vi "Inspect Tell.vi"(8 "Error in":errorcluster, 9 "Msg Attributes":refnum<data-value>, 10 "Alias":string, 11 "TEMPLATE Actor in":refnum<class "TEMPLATE Actor.lvclass">) -> (0 "Error out":errorcluster, 2 "Proceed To Tell":bool=TRUE, 3 "TEMPLATE Actor out":refnum<class "TEMPLATE Actor.lvclass">)   [LabVIEW 2020, in "_Template.lvlib" / "Templates.lvlib" / "TEMPLATE jettl Actor.lvlib" / "TEMPLATE Actor.lvlib" / "TEMPLATE Actor.lvclass"]
uses:
  TEMPLATE Actor.lvclass
  TEMPLATE Actor.lvclass/TEMPLATE Actor.ctl
  jettl/jettl/Actor/Actor.lvclass
  jettl/jettl/Msg/Msg.lvclass
  jettl/jettl/Refs/Refs.lvclass
  jettl/jettl/Relation.ctl
  jettl/jettl/jettl.lvlib
  jettl/jettl/Teller.ctl
  jettl/jettl/Msg Input/Msg Input.lvclass
  jettl/jettl/Msg Output/Msg Output.lvclass
  jettl/jettl/Msg Attributes.ctl
panel:
  # "This front panel should not be manipulated."
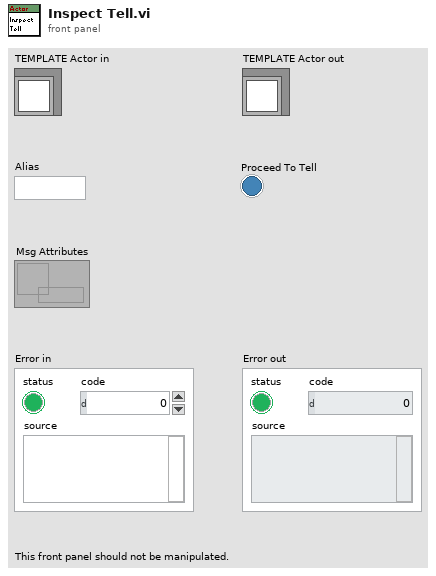
[diagram p1: front panel]
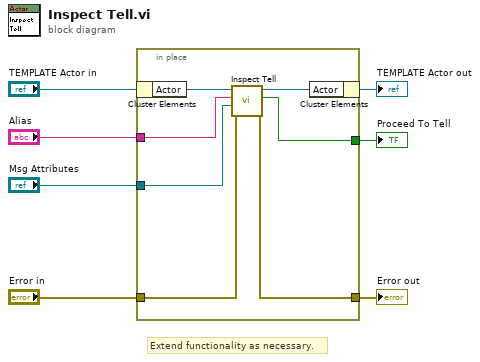
[diagram p0: block diagram]
diagram:
  # "Extend functionality as necessary."
  n1 = in-place {
    in-place-border: "Error in" -> [w11]
    in-place-border: "Msg Attributes" -> [w12]
    in-place-border: [w10] -> w3
    in-place-border: [w9] -> w2
    in-place-border: "Alias" -> [w8]
    n2 = in-place-cluster #1("TEMPLATE Actor in") -> ("Actor"=w14:refnum<data-value>)
    n3 = call-dynamic "Inspect Tell.vi"("Error in"=w11, "Msg Attributes"=w12, "Alias"=w8, "Actor in"=w14) -> ("Error out"=w10:errorcluster, "Proceed To Tell"=w9:bool, "Actor out"=w13:refnum<class "Actor.lvclass">)  [unwired: 5 in]
    n4 = in-place-cluster #1("Actor"=w13) -> (→"TEMPLATE Actor out":refnum<class "TEMPLATE Actor.lvclass">)
  }
  "Proceed To Tell" <- w2
  "Error out" <- w3
